vi "StopGrab.vi"(0 "InputHandle":u64, 1 "error in (no error)":errorcluster) -> (2 "OutputHandle":u64, 3 "GX_STATUS":i32, 4 "error out":errorcluster)   [LabVIEW 2016, in "GxLVLib.lvlib"]
uses:
  GxLVLib.lvlib
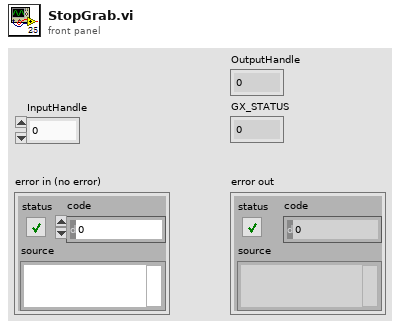
[diagram p1: front panel]
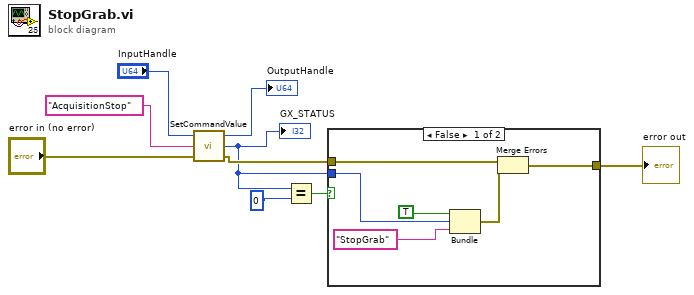
[diagram p0: block diagram]
diagram:
  n1 = call "SetCommandValue.vi"("error in (no error)"="error in (no error)", "strName"="AcquisitionStop", "nInputHandle"="InputHandle") -> ("error out"=w4:errorcluster, "GX_STATUS"=w1:i32, "nOutputHandle"=→"OutputHandle":u64)
  "GX_STATUS" <- w1
  n2 = Equal?(x=w1, y=0) -> (x = y?=w2:bool)
  n3 = case shown="False" w2 {
    tunnel: w4 -> [w15 w16]
    tunnel: [w14 w16] -> w5
    tunnel: w1 -> [w12 _]
    frame False {
      n4 = Bundle(TRUE, "GX_STATUS"=w12, "StopGrab") -> (w13:cluster{bool, "GX_STATUS":i32, string})  [unwired: 1 in]
      n5 = Merge Errors(w15, w13) -> (w14:errorcluster)
    }
    frame True {
    }
  }
  "error out" <- w5
